vi "ConcatenateLV.vi"(8 "error in (no error)":errorcluster, 11 "data":T2[](array[typedef])) -> (0 "error out":errorcluster)   [LabVIEW 2016, in "VCL_2_DSC.lvclass"]
uses:
  VCL_2_DSC.lvclass
  typedefs/TSLtoLV-cluster.ctl
  <userlib>/_OpenG.lib/array/array.llb/Remove Duplicates from 1D Array (String)__ogtk.vi
panel:
  out "Array 2":string[](array[string])
  out "Array":string[](array[string])
  out "XY Graph":T1(graph)
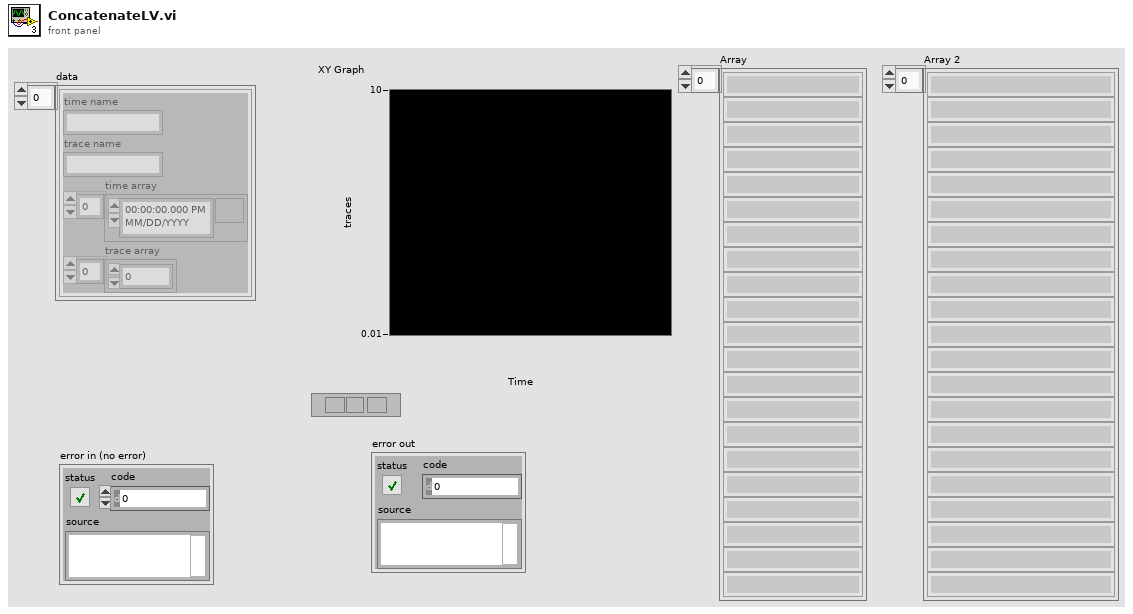
[diagram p1: front panel]
types:
  T1 = cluster{"time array":timestamp[], "trace array":dbl[]}[]
  T2 = typedef "VCL_2_DSC.lvclass/TSLtoLV-cluster.ctl" = cluster{"time name":string, "trace name":string, "time array":timestamp[], "trace array":dbl[]}
  T3 = cluster{"time array":timestamp[], "trace array":dbl[]}
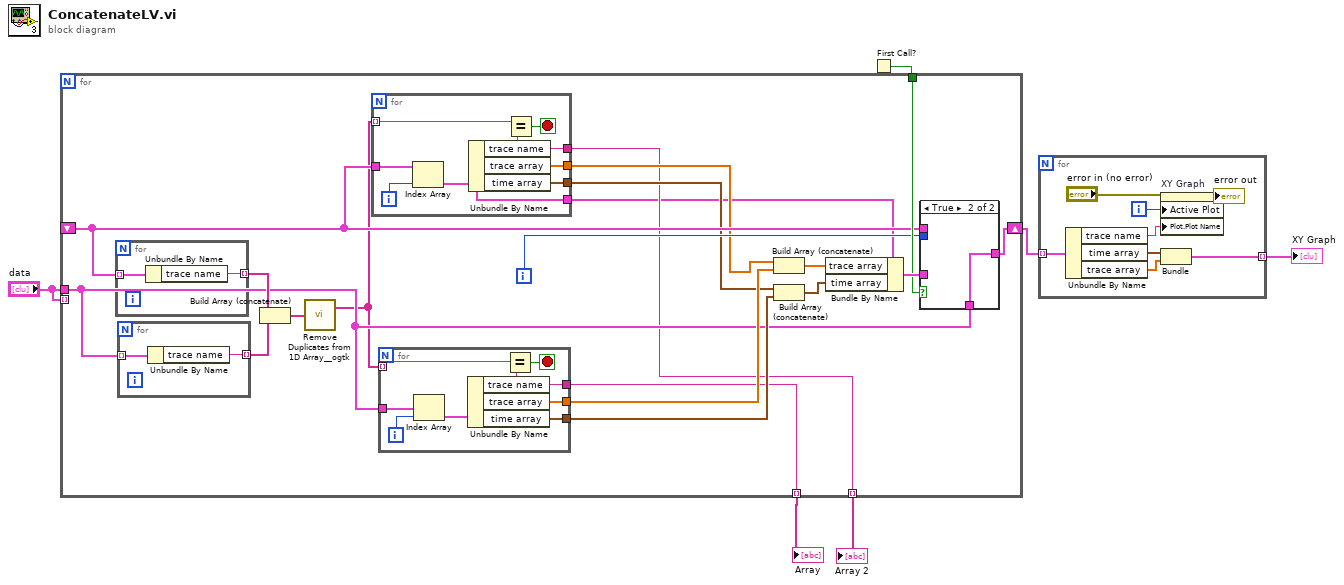
[diagram p0: block diagram]
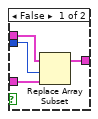
[diagram p2: hidden frame]
diagram:
  n1 = First Call?() -> (First Call?: T/F=w4:bool)
  n2 = for {
    shift-right: [w23] -> w6
    shift-left: _ -> [w12]
    tunnel: "data" -> [_] mode=indexing
    tunnel: "data" -> [w13]
    tunnel: w4 -> [w19]
    tunnel: [w17] -> w2 mode=indexing
    tunnel: [w9] -> w1 mode=indexing
    i -> [w18]
    n3 = for {
      tunnel: w12 -> [w35] mode=indexing
      tunnel: [w34] -> w16 mode=indexing
      n4 = Unbundle By Name(w35) -> ("trace name"=w34:string)
    }
    n5 = for {
      tunnel: w13 -> [w37] mode=indexing
      tunnel: [w36] -> w15 mode=indexing
      n6 = Unbundle By Name(w37) -> ("trace name"=w36:string)
    }
    n7 = Build Array (concatenate)(w16, w15) -> (w14:string[])
    n8 = call-poly <userlib>:"Remove Duplicates from 1D Array__ogtk.vi"("Input Array"=w14) -> ("Output Array"=w7:string[])  [unwired: 1 out]
    n9 = for {
      tunnel: [w33] -> w11
      tunnel: [w32] -> w10
      tunnel: w12 -> [w27]
      tunnel: [w30] -> w9
      tunnel: [w26] -> w8
      tunnel: w7 -> [w29] mode=indexing
      i -> [w28]
      stop <- w31 stop-if-true
      n10 = Index Array(array=w27, index=w28) -> (element=w26:T2)
      n11 = Unbundle By Name(w26) -> ("trace name"=w30:string, "trace array"=w33:dbl[], "time array"=w32:timestamp[])
      n12 = Equal?(x=w29, y=w30) -> (x = y?=w31:bool)
    }
    n13 = for {
      tunnel: [w45] -> w22
      tunnel: [w44] -> w21
      tunnel: w13 -> [w39]
      tunnel: w7 -> [w42] mode=indexing
      tunnel: [w41] -> w17
      i -> [w40]
      stop <- w43 stop-if-true
      n14 = Index Array(array=w39, index=w40) -> (element=w38:T2)
      n15 = Unbundle By Name(w38) -> ("trace name"=w41:string, "trace array"=w45:dbl[], "time array"=w44:timestamp[])
      n16 = Equal?(x=w42, y=w41) -> (x = y?=w43:bool)
    }
    n17 = Build Array (concatenate)(w11, w22) -> (w25:dbl[])
    n18 = Build Array (concatenate)(w10, w21) -> (w20:timestamp[])
    n19 = Bundle By Name(cluster=w8, "trace array"=w25, "time array"=w20) -> (w24:T2)
    n20 = case shown="True" w19 {
      tunnel: w18 -> [w49 _]
      tunnel: w24 -> [w46 _]
      tunnel: [w48 w50] -> w23
      tunnel: w12 -> [w47 _]
      tunnel: w13 -> [_ w50]
      frame False {
        n21 = Replace Array Subset(array=w47, new element=w46, index=w49) -> (w48:T2[])
      }
      frame True {
      }
    }
  }
  "Array" <- w2
  "Array 2" <- w1
  n22 = for {
    tunnel: w6 -> [w58] mode=indexing
    tunnel: [w55] -> w5 mode=indexing
    i -> [w53]
    n23 = Unbundle By Name(w58) -> ("trace name"=w54:string, "time array"=w57:timestamp[], "trace array"=w56:dbl[])
    n24 = property on="XY Graph" class="XYGraph (strict)"(error in="error in (no error)", "Active Plot"=w53, "Plot.Plot Name"=w54) -> (error out=→"error out":errorcluster)  [unwired: 1 in, 1 out]
    n25 = Bundle("time array"=w57, "trace array"=w56) -> (w55:T3)  [unwired: 1 in]
  }
  "XY Graph" <- w5
